vi "Test FINS3-E BusB Data Acquisition and Decoding API.vi"() -> ()   [LabVIEW 2016]
doc: "FINS3-E BusB Data Acquisition and Decoding API Tester."
uses:
  BusB Typedef.ctl
  FINS3-E BusB Data Acquisition and Decoding.lvlib
panel:
  in  "Initialize FINS for Qualification":bool
  in  "Initialize FINS for FTR":bool
  in  "Initialize FINS":bool
  out "Pitch Rate":dbl(graph)
  out "BusB":T1
  out "BusB Raw Data":u8[](array[numeric])
  in  "Start Acquiring":bool
  in  "Settings":bool
  out "BusB Visa Resource":refnum<visa-resource-name>
  out "Acquiring?":bool
  in  "Stop Acquiring":bool
  in  "Show Block Diagram":bool
  in  "Stop Module":bool
  in  "Start Module":bool
  in  "Hide Module Panel":bool
  in  "Show Module Panel":bool
  out "Status":string
  out "Module Running?":bool
  # "This VI tests the API for the Module."
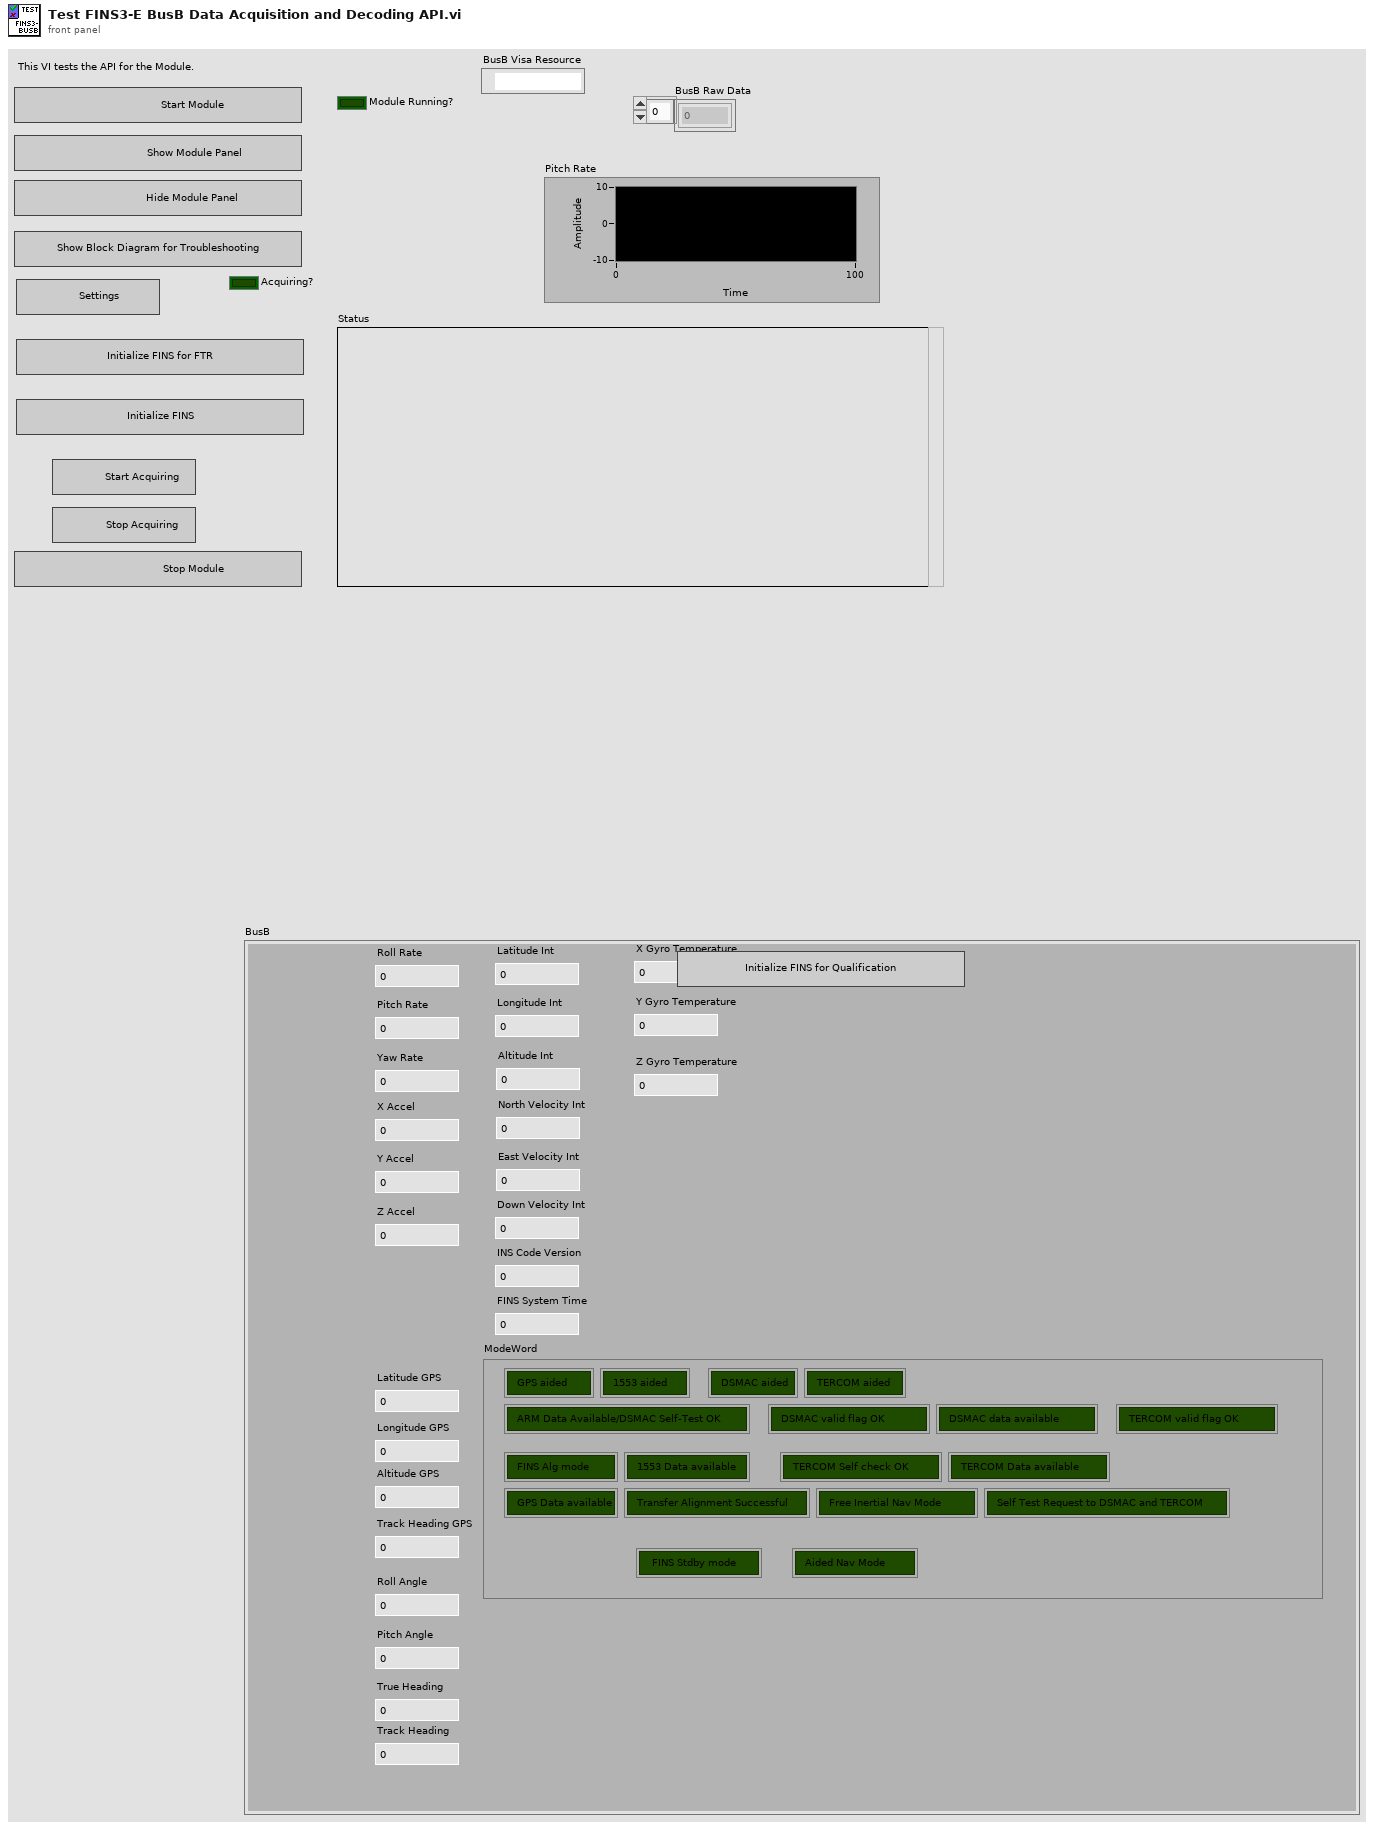
[diagram p1: front panel]
types:
  T1 = typedef "FINS3-E (Rx-I) Library.lvlib/FINS3-E BusB Data Acquisition and Decoding.lvlib/BusB Typedef.ctl" = cluster{"Pitch Rate":dbl, "Roll Rate":dbl, "Roll Angle":dbl, "Yaw Rate":dbl, "True Heading":dbl, "Pitch Angle":dbl, "Y Accel":dbl, "X Accel":dbl, "Z Accel":dbl, "X Gyro Temperature":dbl, "Longitude GPS":dbl, "Latitude GPS":dbl, "Altitude GPS":dbl, "Track Heading GPS":dbl, "Longitude Int":dbl, "Latitude Int":dbl, "Altitude Int":dbl, "FINS System Time":dbl, "East Velocity Int":dbl, "North Velocity Int":dbl, "INS Code Version":dbl, "ModeWord":cluster{"FINS Alg mode":bool, "GPS Data available":bool, "1553 Data available":bool, "Transfer Alignment Successful":bool, "TERCOM Self check OK":bool, "Free Inertial Nav Mode":bool, "TERCOM Data available":bool, "Self Test Request to DSMAC and TERCOM":bool, "ARM Data Available/DSMAC Self-Test OK":bool, "DSMAC valid flag OK":bool, "DSMAC data available":bool, "TERCOM valid flag OK":bool, "GPS aided":bool, "1553 aided":bool, "DSMAC aided":bool, "TERCOM aided":bool, "Aided Nav Mode":bool, " FINS Stdby mode":bool}, "Down Velocity Int":dbl, "Track Heading":dbl, "Y Gyro Temperature":dbl, "Z Gyro Temperature":dbl}
  T2 = typedef "FINS3-E (Rx-I) Library.lvlib/FINS3-E BusB Data Acquisition and Decoding.lvlib/Broadcast Events--cluster.ctl" = cluster{"Module Did Init":refnum<user-event>, "Status Updated":refnum<user-event>, "Error Reported":refnum<user-event>, "Module Did Stop":refnum<user-event>, "Update Module Execution Status":refnum<user-event>, "Acquisition Stopped":refnum<user-event>, "BusB Raw Data":refnum<user-event>, "BusB Decoded Data Updated":refnum<user-event>, "Acquisition Started":refnum<user-event>, "Read Timeout Error Generation":refnum<user-event>}
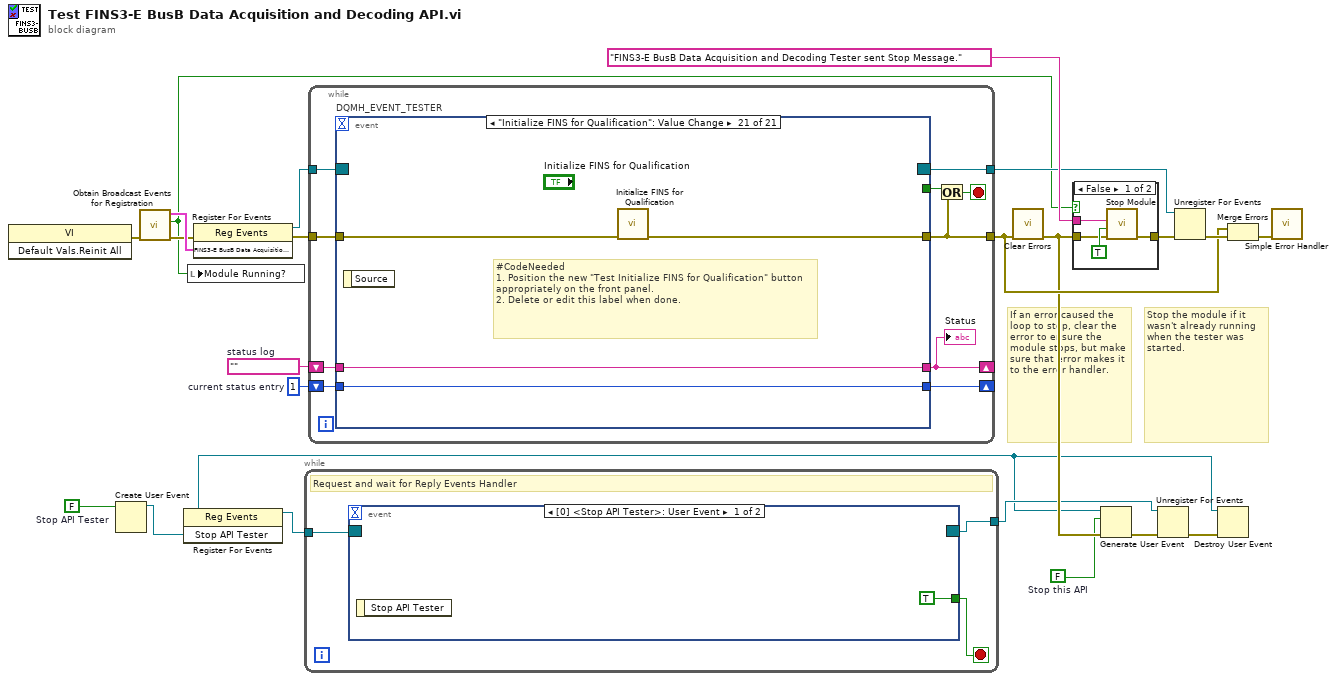
[diagram p0: block diagram]
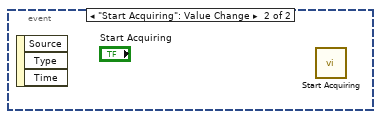
[diagram p2: hidden frame]
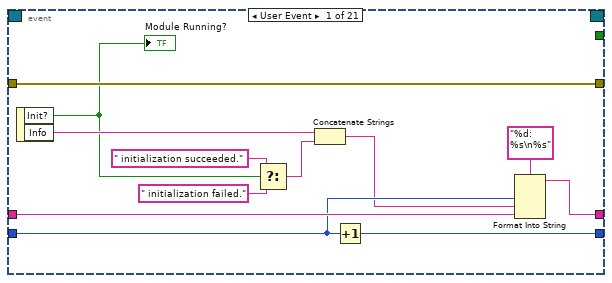
[diagram p4: hidden frame]
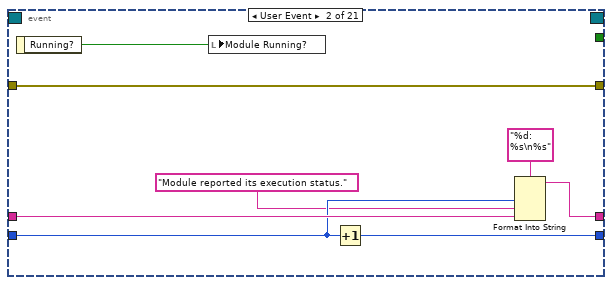
[diagram p5: hidden frame]
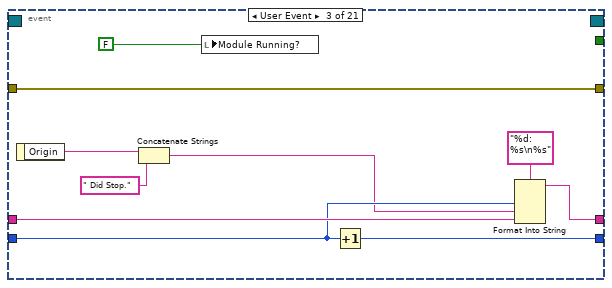
[diagram p6: hidden frame]
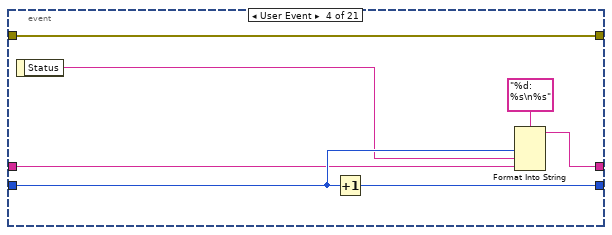
[diagram p7: hidden frame]
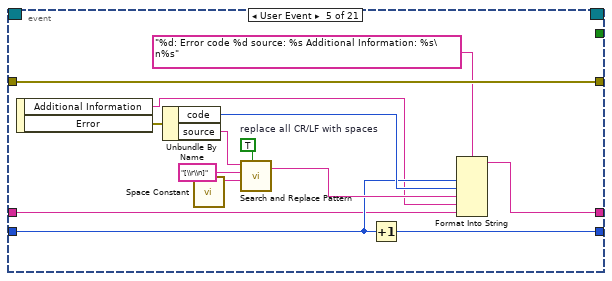
[diagram p8: hidden frame]
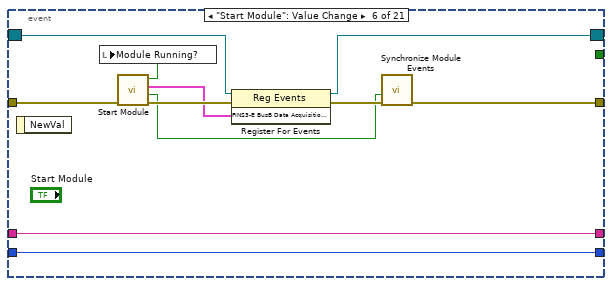
[diagram p9: hidden frame]
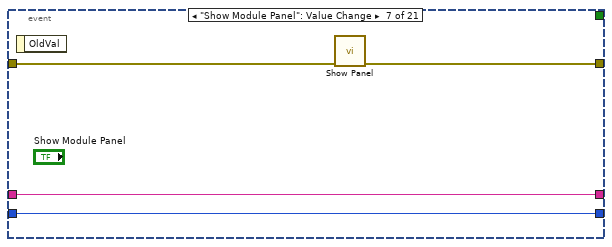
[diagram p10: hidden frame]
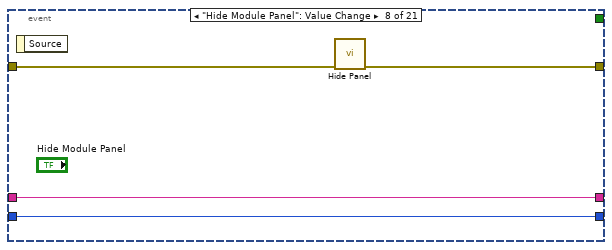
[diagram p11: hidden frame]
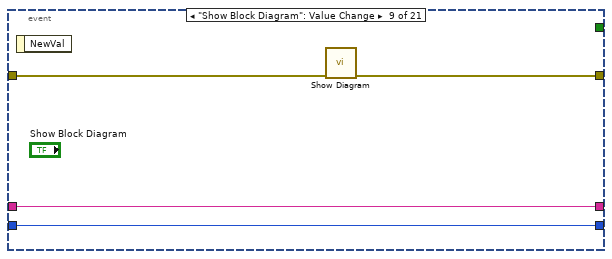
[diagram p12: hidden frame]
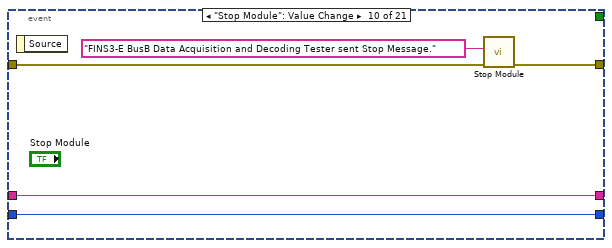
[diagram p13: hidden frame]
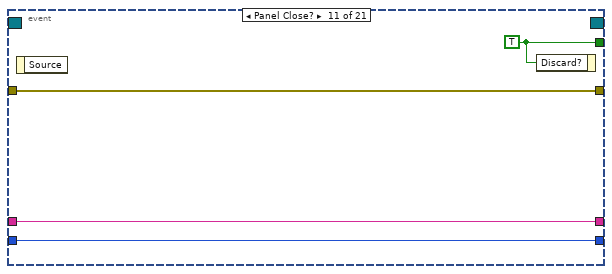
[diagram p14: hidden frame]
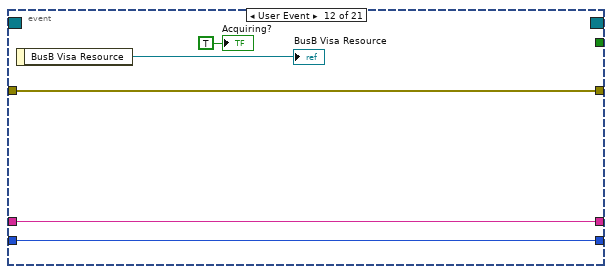
[diagram p15: hidden frame]
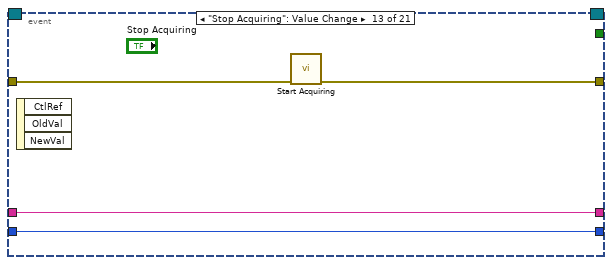
[diagram p16: hidden frame]
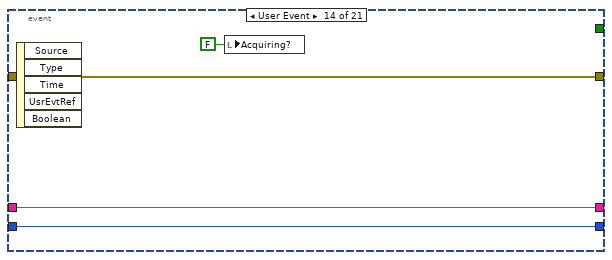
[diagram p17: hidden frame]
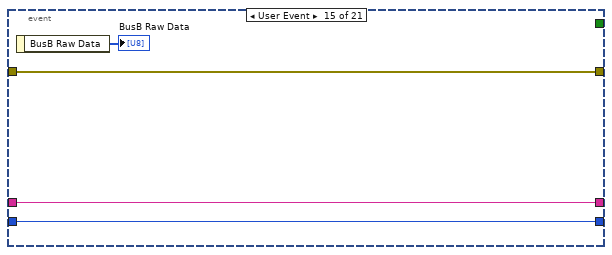
[diagram p18: hidden frame]
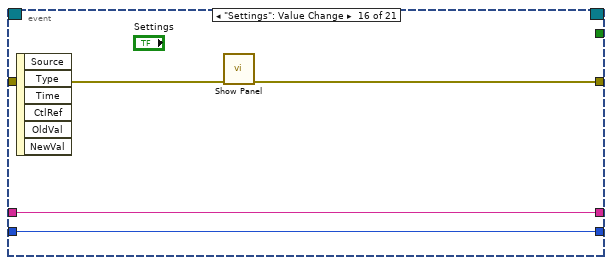
[diagram p19: hidden frame]
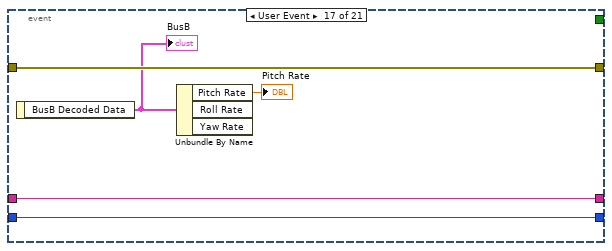
[diagram p20: hidden frame]
diagram:
  w1 = FALSE  # Stop this API
  w2 = FALSE  # Stop API Tester
  w18 = 1  # current status entry
  w19 = ""  # status log
  # "Stop the module if it wasn't already running when the tester was started."
  # "If an error caused the loop to stop, clear the error to ensure the module stops, but make sure that error makes it to the error handler."
  n1 = invoke class="VI" method="Default Vals.Reinit All"() -> (error out=w11:errorcluster)  [unwired: 3 in, 2 out]
  n2 = Create User Event(user event datatype=w2) -> (user event=w3:refnum<user-event>)  [unwired: 1 in, 1 out]
  n3 = call "Obtain Broadcast Events for Registration.vi"("error in (no error)"=w11) -> ("error out"=w10:errorcluster, "Already running?"=w9:bool, "FINS3-E BusB Data Acquisition and Decoding Broadcast Events"=w16:T2)  [unwired: 8 in]
  n4 = register-events(w3) -> (reference out=w8:refnum<event-registration>)  [unwired: 2 in, 1 out]
  n5 = local write "Module Running?"(w9) -> ()
  n6 = register-events(error in=w10, w16) -> (reference out=w15:refnum<event-registration>, error out=w17:errorcluster)  [unwired: 1 in]
  n7 = while {
    tunnel: w8 -> [w25]
    tunnel: [w24] -> w4
    stop <- w23 stop-if-true
    # "Request and wait for Reply Events Handler"
    n8 = event shown="[0] <Stop API Tester>: User Event" {
      selector: w25 -> [_ _]
      dyn-events: [_ _] -> w24
      timeout: _ -> [_ _]
      tunnel: [TRUE _] -> w23
      event User Event {
        n9 = event-data() -> ()  [unwired: 1 in, 1 out]
      }
      event "Start Acquiring": Value Change {
        n10 = event-data() -> ()  [unwired: 1 in, 3 out]
        n11 = call "Start Acquiring.vi"() -> ()  [unwired: 9 in, 3 out]
      }
    }
  }
  n12 = while {
    tunnel: w15 -> [w36]
    tunnel: [w27] -> w12
    shift-right: [w31] -> _
    shift-left: w19 -> [w33]
    shift-right: [w32] -> _
    shift-left: w18 -> [w34]
    tunnel: w17 -> [w29]
    tunnel: [w28] -> w14
    stop <- w30 stop-if-true
    n13 = event "DQMH_EVENT_TESTER" shown="[20] \"Initialize FINS for Qualification\": Value Change" {
      selector: w36 -> [_ _ _ _ _ w92 _ _ _ _ _ _ _ _ _ _ _ _ _ _ _]
      dyn-events: [_ _ _ _ _ w91 _ _ _ _ _ _ _ _ _ _ _ _ _ _ _] -> w28
      timeout: _ -> [_ _ _ _ _ _ _ _ _ _ _ _ _ _ _ _ _ _ _ _ _]
      tunnel: [_ _ _ _ _ _ _ _ _ _ w119 _ _ _ _ _ _ _ _ _ _] -> w35
      tunnel: [w48 w50 w57 w67 w87 w90 w102 w106 w107 w113 w116 w124 w125 w132 w136 w137 w145 w146 w152 w153 w157] -> w27
      tunnel: w34 -> [w45 w54 w64 w70 w77 w95 w100 w104 w108 w114 w117 w122 w126 w130 w134 w139 w143 w147 w150 w154 w158]
      tunnel: w33 -> [w46 w55 w65 w69 w75 w96 w101 w105 w109 w115 w118 w123 w127 w131 w135 w140 w144 w148 w151 w155 w159]
      tunnel: [w43 w52 w62 w71 w78 w96 w101 w105 w109 w115 w118 w123 w127 w131 w135 w140 w144 w148 w151 w155 w159] -> w31
      tunnel: [w44 w53 w63 w73 w76 w95 w100 w104 w108 w114 w117 w122 w126 w130 w134 w139 w143 w147 w150 w154 w158] -> w32
      tunnel: w29 -> [w48 w50 w57 w67 w87 w89 w99 w103 w110 w111 w116 w124 w128 w132 w136 w138 w145 w149 w152 w156 w160]
      event User Event {
        n14 = event-data() -> ("Init?"=w40:bool, "Info"=w42:string)  [unwired: 1 in]
        "Module Running?" <- w40
        n15 = Select(t=" initialization succeeded.", s=w40, f=" initialization failed.") -> (s? t:f=w37:string)
        n16 = Concatenate Strings(w42, w37) -> (w41:string)
        n17 = Increment(x=w45) -> (x+1=w44:i32)
        n18 = Format Into String(format string="%d: %s\n%s", w45, w41, w46) -> (resulting string=w43:string)  [unwired: 2 in, 1 out]
      }
      event User Event {
        n19 = event-data() -> ("Running?"=w49:bool)  [unwired: 1 in]
        n20 = local write "Module Running?"(w49) -> ()
        n21 = Increment(x=w54) -> (x+1=w53:i32)
        n22 = Format Into String(format string="%d: %s\n%s", w54, "Module reported its execution status.", w55) -> (resulting string=w52:string)  [unwired: 2 in, 1 out]
      }
      event User Event {
        n23 = event-data() -> ("Origin"=w61:string)  [unwired: 1 in]
        n24 = Concatenate Strings(w61, " Did Stop.") -> (w60:string)
        n25 = local write "Module Running?"(FALSE ("Module Did Init?")) -> ()
        n26 = Increment(x=w64) -> (x+1=w63:i32)
        n27 = Format Into String(format string="%d: %s\n%s", w64, w60, w65) -> (resulting string=w62:string)  [unwired: 2 in, 1 out]
      }
      event User Event {
        n28 = event-data() -> ("Status"=w68:string)  [unwired: 1 in]
        n29 = Increment(x=w70) -> (x+1=w73:i32)
        n30 = Format Into String(format string="%d: %s\n%s", w70, w68, w69) -> (resulting string=w71:string)  [unwired: 2 in, 1 out]
      }
      event User Event {
        w83 = TRUE  # replace all CR/LF with spaces
        n31 = event-data() -> ("Additional Information"=w74:string, "Error"=w79:errorcluster)  [unwired: 1 in]
        n32 = Unbundle By Name(w79) -> ("code"=w80:i32, "source"=w81:string)
        n33 = call <vilib>:"Space Constant.vi"() -> ("String"=w84:string)
        n34 = call <vilib>:"Search and Replace Pattern.vi"("string"=w81, "regular expression (\"\")"="[\\r\\n]" ("regular expression (\"\")"), "replace string (\"\")"=w84, "replace all? (F)"=w83) -> ("result string"=w82:string)  [unwired: 1 in, 1 out]
        n35 = Increment(x=w77) -> (x+1=w76:i32)
        n36 = Format Into String(format string="%d: Error code %d source: %s Additional Information: %s\n%s", w77, w80, w82, w74, w75) -> (resulting string=w78:string)  [unwired: 2 in, 1 out]
      }
      event "Start Module": Value Change {
        n37 = event-data() -> ()  [unwired: 1 in, 1 out]
        n38 = call "Start Module.vi"("error in (no error)"=w89) -> ("error out"=w97:errorcluster, "Wait for Event Sync?"=w94:bool, "FINS3-E BusB Data Acquisition and Decoding Broadcast Events"=w93:T2, "Module Was Already Running?"=w88:bool)  [unwired: 7 in]
        n39 = local write "Module Running?"(w88) -> ()
        n40 = register-events(reference=w92, error in=w97, w93) -> (reference out=w91:refnum<event-registration>, error out=w98:errorcluster)
        n41 = call "Synchronize Module Events.vi"("error in (no error)"=w98, "Wait for Event Sync?"=w94) -> ("error out"=w90:errorcluster)  [unwired: 9 in]
      }
      event "Show Module Panel": Value Change {
        n42 = event-data() -> ()  [unwired: 1 in, 1 out]
        n43 = call "Show Panel.vi"("error in (no error)"=w99) -> ("error out"=w102:errorcluster)  [unwired: 10 in]
      }
      event "Hide Module Panel": Value Change {
        n44 = event-data() -> ()  [unwired: 1 in, 1 out]
        n45 = call "Hide Panel.vi"("error in (no error)"=w103) -> ("error out"=w106:errorcluster)  [unwired: 10 in]
      }
      event "Show Block Diagram": Value Change {
        n46 = event-data() -> ()  [unwired: 1 in, 1 out]
        n47 = call "Show Diagram.vi"("error in (no error)"=w110) -> ("error out"=w107:errorcluster)  [unwired: 10 in]
      }
      event "Stop Module": Value Change {
        n48 = event-data() -> ()  [unwired: 1 in, 1 out]
        n49 = call "Stop Module.vi"("error in (no error)"=w111, "Origin"="FINS3-E BusB Data Acquisition and Decoding Tester sent Stop Message.") -> ("error out"=w113:errorcluster)  [unwired: 9 in]
      }
      event Panel Close? {
        w119 = TRUE ("Discard?")
        n50 = event-data() -> ()  [unwired: 1 in, 1 out]
        n51 = event-data("Discard?"=w119) -> ()  [unwired: 1 in, 1 out]
      }
      event User Event {
        n52 = event-data() -> ("BusB Visa Resource"=→"BusB Visa Resource":refnum<visa-resource-name>)  [unwired: 1 in]
        "Acquiring?" <- TRUE ("Acquiring?")
      }
      event "Stop Acquiring": Value Change {
        n53 = event-data() -> ()  [unwired: 1 in, 3 out]
        n54 = call "Start Acquiring.vi"("error in (no error)"=w128) -> ("error out"=w125:errorcluster)  [unwired: 8 in, 2 out]
      }
      event User Event {
        n55 = event-data() -> ()  [unwired: 1 in, 5 out]
        n56 = local write "Acquiring?"(FALSE ("Acquiring?")) -> ()
      }
      event User Event {
        n57 = event-data() -> ("BusB Raw Data"=→"BusB Raw Data":u8[])  [unwired: 1 in]
      }
      event "Settings": Value Change {
        n58 = event-data() -> ()  [unwired: 1 in, 6 out]
        n59 = call "Show Panel.vi"("error in (no error)"=w138) -> ("error out"=w137:errorcluster)  [unwired: 10 in]
      }
      event User Event {
        n60 = event-data() -> ("BusB Decoded Data"=w142:T1)  [unwired: 1 in]
        "BusB" <- w142
        n61 = Unbundle By Name(w142) -> ("Pitch Rate"=→"Pitch Rate":dbl)  [unwired: 2 out]
      }
      event "Initialize FINS": Value Change {
        # "#CodeNeeded\n1. Position the new \"Test Initialize FINS\" button appropriately on the front panel.\n2. Delete or edit this label when done."
        n62 = event-data() -> ()  [unwired: 1 in, 1 out]
        n63 = call "Initialize FINS.vi"("error in (no error)"=w149) -> ("error out"=w146:errorcluster)  [unwired: 10 in]
      }
      event User Event {
        # "#CodeNeeded\n1. Process the event data sent by the \"Read Timeout Error Generation\" broadcast event.\n2. Delete or edit this label when done."
        n64 = event-data() -> ()  [unwired: 1 in, 5 out]
      }
      event "Initialize FINS for FTR": Value Change {
        # "#CodeNeeded\n1. Position the new \"Test Initialize FINS for FTR\" button appropriately on the front panel.\n2. Delete or edit this label when done."
        n65 = event-data() -> ()  [unwired: 1 in, 1 out]
        n66 = call "Initialize FINS for FTR.vi"("error in (no error)"=w156) -> ("error out"=w153:errorcluster)  [unwired: 10 in]
      }
      event "Initialize FINS for Qualification": Value Change {
        # "#CodeNeeded\n1. Position the new \"Test Initialize FINS for Qualification\" button appropriately on the front panel.\n2. Delete or edit this label when done."
        n67 = event-data() -> ()  [unwired: 1 in, 1 out]
        n68 = call "Initialize FINS for Qualification.vi"("error in (no error)"=w160) -> ("error out"=w157:errorcluster)  [unwired: 10 in]
      }
    }
    "Status" <- w31
    n69 = Or(x=w35, y=w27) -> (x .or. y?=w30:bool)
  }
  n70 = call <vilib>:"Clear Errors.vi"("error in (no error)"=w12) -> ("error out"=w5:errorcluster)  [unwired: 5 in, 1 out]
  n71 = case shown="False" w9 {
    tunnel: [w164 w165] -> w21
    tunnel: "FINS3-E BusB Data Acquisition and Decoding Tester sent Stop Message." ("Origin") -> [w163 _]
    tunnel: w5 -> [w161 w165]
    frame False {
      n72 = call "Stop Module.vi"("error in (no error)"=w161, "Wait for Module to Stop? (F)"=TRUE ("Wait for Module to stop?"), "Origin"=w163) -> ("error out"=w164:errorcluster)  [unwired: 8 in]
    }
    frame True {
    }
  }
  n73 = Generate User Event(user event=w3, event data cluster=w1, error in=w5) -> (error out=w6:errorcluster)  [unwired: 1 in, 1 out]
  n74 = Unregister For Events(event registration refnum=w4, error in=w6) -> (error out=w7:errorcluster)
  n75 = Unregister For Events(event registration refnum=w14, error in=w21) -> (error out=w22:errorcluster)
  n76 = Destroy User Event(user event=w3, error in=w7) -> ()  [unwired: 1 out]
  n77 = Merge Errors(w12, w22) -> (w13:errorcluster)
  n78 = call <vilib>:"Simple Error Handler.vi"("error in (no error)"=w13) -> ()  [unwired: 4 in, 5 out]
